vi "CreatePrivateEvents.vi"(8 "error in (no error)":errorcluster, 11 "SMO.BasicByRef":refnum<class "SMO.BasicByRef.lvclass">) -> (0 "error out":errorcluster, 3 "SMO.BasicByRef out":refnum<class "SMO.BasicByRef.lvclass">)   [LabVIEW 2013, in "SMO.BasicByRef.lvclass"]
doc: "JKI State Machine Objects (SMO) 1.0.2.13\nJKI - JKI\nCopyright (c) 2016, JKI"
uses:
  SMO.BasicByRef.lvclass
  <vilib>/JKI/JKI SMO/SMO/SMO.lvclass
  SMO.BasicByRef.lvclass/SMO.BasicByRef.ctl
  Typedefs/NewValueEvent--Cluster.ctl
panel:
  # "For instructions on how to use the JKI State Machine Objects, examples and video tutorials, visit:\nhttp://jki.net/state-machine-objects/\n\nJKI State Machine Objects™\nhttp://jki.net/state-machine-objects/\nCopyright (C) 2005-2015, JKI <info@jki.net>\nALL RIGHTS RESERVED"
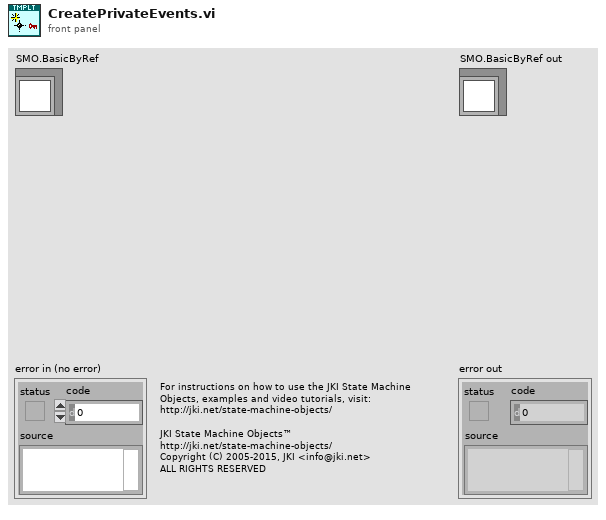
[diagram p1: front panel]
types:
  T1 = typedef "SMO.BasicByRef.lvclass/PrivateData--Ref.ctl" = refnum<data-value>
  T2 = typedef "SMO.BasicByRef.lvclass/NewValueEvent--Cluster.ctl" = cluster{"Data":string}
  T3 = typedef "SMO.BasicByRef.lvclass/PrivateData--Cluster.ctl" = cluster{"Public Events":T4, "Protected Events":T5, "Private Events":T6, "Value":T7}
  T4 = typedef "SMO.BasicByRef.lvclass/PublicEvents--Cluster.ctl" = cluster{"Data Changed":refnum<user-event>}
  T5 = typedef "SMO.BasicByRef.lvclass/ProtectedEvents--Cluster.ctl" = cluster{"API_Template":refnum<user-event>}
  T6 = typedef "SMO.BasicByRef.lvclass/PrivateEvents--Cluster.ctl" = cluster{"New Value":refnum<user-event>}
  T7 = typedef "SMO.BasicByRef.lvclass/Value.ctl" = string
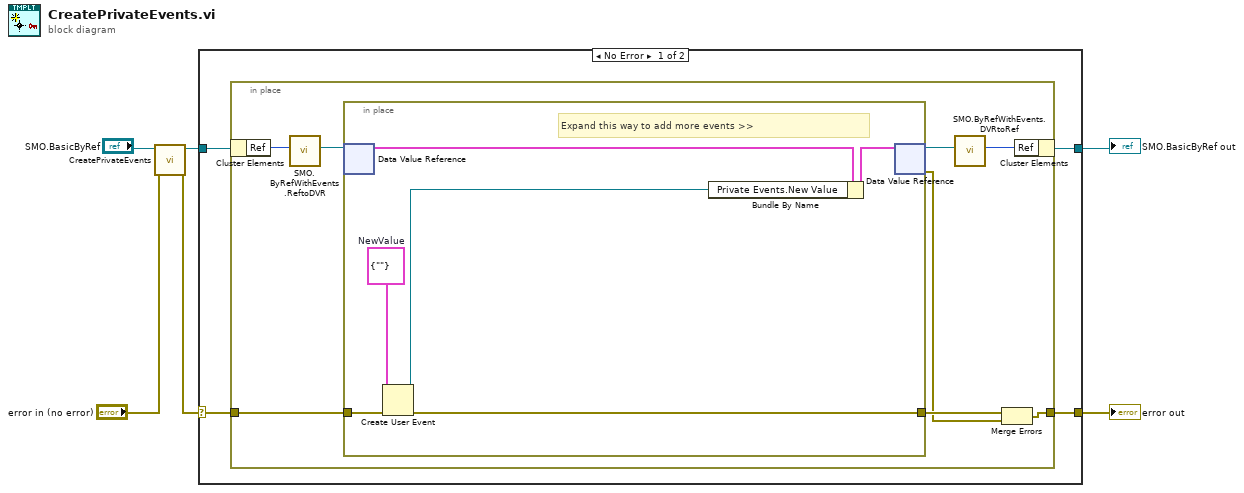
[diagram p0: block diagram]
diagram:
  n1 = call-parent "CreatePrivateEvents.vi"("error in (no error)"="error in (no error)", "SMO"="SMO.BasicByRef") -> ("error out"=w5:errorcluster, "SMO out"=w6:refnum<class "SMO.BasicByRef.lvclass">)  [unwired: 8 in]
  n2 = case shown="No Error" w5 {
    selector: w5 -> [w8 w26]
    tunnel: [w7 w26] -> w1
    tunnel: [w9 w25] -> w3
    tunnel: w6 -> [w10 w25]
    frame No Error {
      n3 = in-place {
        in-place-border: w8 -> [w18]
        in-place-border: [w15] -> w7
        n4 = in-place-cluster #1(w10) -> ("Ref"=w14:u32)
        n5 = call "SMO.ByRefWithEvents.ReftoDVR.vi"("Ref"=w14) -> ("Ref"=w13:T1)  [unwired: 10 in]
        n6 = in-place {
          in-place-border: w18 -> [w22]
          in-place-border: [w23] -> w17
          w19 = T2 {"Data"=""}  # NewValue
          # "Expand this way to add more events >>"
          n7 = in-place-dvr #2(w13) -> (w21:T3)  [unwired: 1 out]
          n8 = Create User Event(user event datatype=w19, error in=w22) -> (user event=w20:refnum<user-event>, error out=w23:errorcluster)
          n9 = Bundle By Name(cluster=w21, "Private Events.New Value"=w20) -> (w24:T3)
          n10 = in-place-dvr #2(w24) -> (w12:T1, w16:errorcluster)
        }
        n11 = call "SMO.ByRefWithEvents.DVRtoRef.vi"("Ref"=w12) -> ("Ref"=w11:u32)  [unwired: 10 in]
        n12 = Merge Errors(w17, w16) -> (w15:errorcluster)
        n13 = in-place-cluster #1("Ref"=w11) -> (w9:refnum<class "SMO.BasicByRef.lvclass">)
      }
    }
    frame Error {
    }
  }
  "error out" <- w1
  "SMO.BasicByRef out" <- w3
